vi "Event Handler.vi"(8 "error in (no error)":errorcluster, 11 "Data Grid in":refnum<class "Data Grid.lvclass">) -> (0 "error out":errorcluster, 3 "Data Grid out":refnum<class "Data Grid.lvclass">)   [LabVIEW 2013, in "Table Manager.lvlib" / "Data Grid.lvclass"]
uses:
  Data Grid.lvclass
  Data Grid.lvclass/Data Grid.ctl
  Table Manager.lvlib
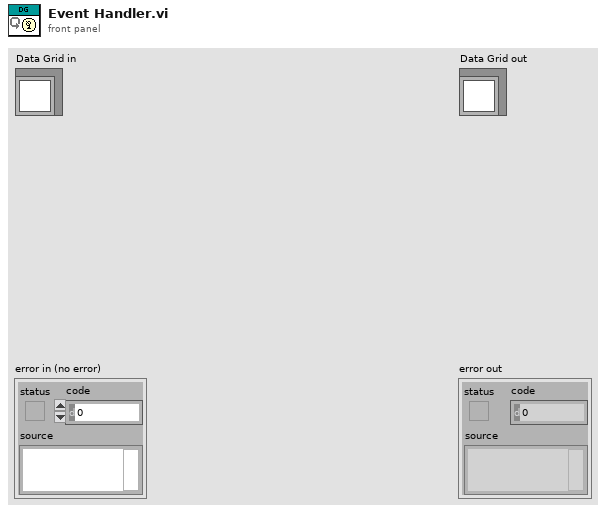
[diagram p1: front panel]
types:
  T1 = typedef "NISE_CEF_Node.lvclass/RefreshUIEvent.ctl" = refnum<user-event>
  T2 = cluster{"Data Grid":refnum<event-registration>, "Node Events":refnum<event-registration>}
  T3 = typedef "Table Manager.lvlib/Table Manager.lvclass/object ref.ctl" = cluster{"engine":refnum<data-value>, "Node Ref":refnum<data-value>}
  T4 = typedef "control module editor.lvclass/dialog output action.ctl" = enum16{"Tag Created", "Tag Selected", "Set Default", "disconnect"}
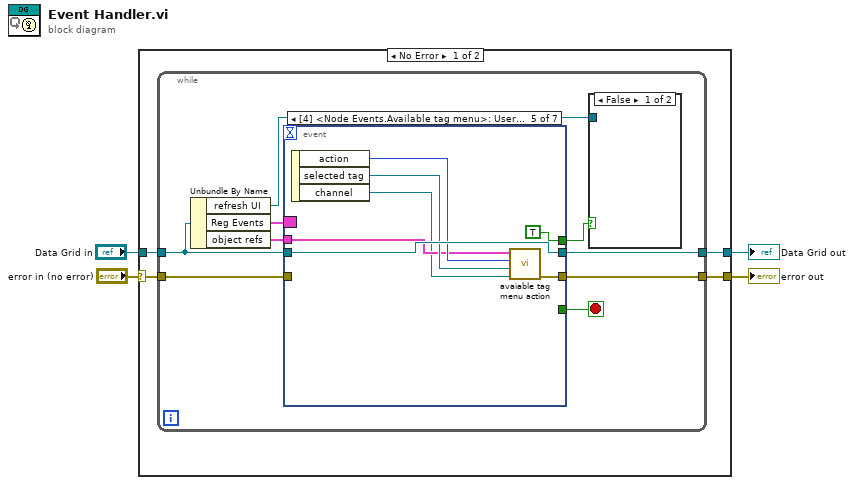
[diagram p0: block diagram]
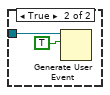
[diagram p2: hidden frame]
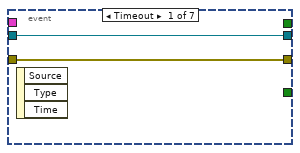
[diagram p3: hidden frame]
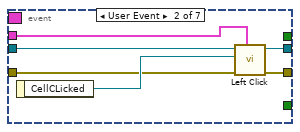
[diagram p4: hidden frame]
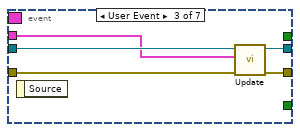
[diagram p5: hidden frame]
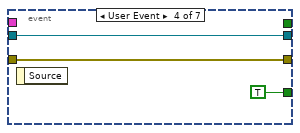
[diagram p6: hidden frame]
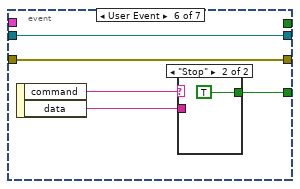
[diagram p7: hidden frame]
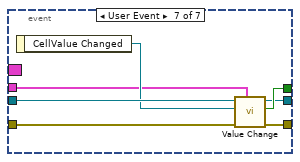
[diagram p9: hidden frame]
diagram:
  n1 = case shown="No Error" "error in (no error)" {
    selector: "error in (no error)" -> [w6 w56]
    tunnel: [w8 w57] -> w3
    tunnel: "Data Grid in" -> [w7 w57]
    tunnel: [w5 w56] -> w1
    frame No Error {
      n2 = while {
        tunnel: [w17] -> w8
        tunnel: w7 -> [w16]
        tunnel: w6 -> [w14]
        tunnel: [w13] -> w5
        stop <- w11 stop-if-true
        n3 = Unbundle By Name(w16) -> ("refresh UI"=w9:T1, "Reg Events"=w15:T2, "object refs"=w12:T3)
        n4 = event shown="[4] <Node Events.Available tag menu>: User Event" {
          selector: w15 -> [_ _ _ _ _ _ _]
          dyn-events: _ -> [_ _ _ _ _ _ _]
          timeout: _ -> [_ _ _ _ _ _ _]
          tunnel: [w21 w26 w31 w34 w42 w47 w53] -> w17
          tunnel: w16 -> [w21 w27 w32 w34 w42 w47 w54]
          tunnel: w14 -> [w20 w24 w30 w33 _ w46 w52]
          tunnel: [w20 w23 w29 w33 w37 w46 w51] -> w13
          tunnel: w12 -> [_ w22 w28 _ w39 _ w49]
          tunnel: [_ _ _ TRUE _ w43 _] -> w11
          tunnel: [_ _ _ _ TRUE _ w55] -> w10
          event Timeout {
            n5 = event-data() -> ()  [unwired: 1 in, 3 out]
          }
          event User Event {
            n6 = event-data() -> ("CellCLicked"=w25:refnum<class "Abstract EVENT.lvclass">)  [unwired: 1 in]
            n7 = call-dynamic "Left Click.vi"("object refs"=w22, "error in (no error)"=w24, "Event data"=w25, "Data Grid in"=w27) -> ("error out"=w23:errorcluster, "Data Grid out"=w26:refnum<class "Data Grid.lvclass">)  [unwired: 5 in, 1 out]
          }
          event User Event {
            n8 = event-data() -> ()  [unwired: 1 in, 1 out]
            n9 = call-dynamic "Update.vi"("error in"=w30, "object ref in"=w28, "Data Grid in"=w32) -> ("error out"=w29:errorcluster, "Data Grid out"=w31:refnum<class "Data Grid.lvclass">)  [unwired: 6 in, 1 out]
          }
          event User Event {
            n10 = event-data() -> ()  [unwired: 1 in, 1 out]
          }
          event User Event {
            n11 = event-data() -> ("action"=w40:T4, "selected tag"=w41:refnum<class "tag descriptor.lvclass">, "channel"=w38:refnum<class "TBM channel.lvclass">)  [unwired: 1 in]
            n12 = call "avaiable tag menu action.vi"("channel"=w38, "selected tag"=w41, "action"=w40, "object ref"=w39) -> ("error out"=w37:errorcluster)  [unwired: 6 in, 1 out]
          }
          event User Event {
            n13 = event-data() -> ("command"=w45:string, "data"=w44:string)  [unwired: 1 in]
            n14 = case shown="\"Stop\"" w45 {
              tunnel: [_ TRUE] -> w43
              tunnel: w44 -> [_ _]
              frame Default {
              }
              frame "Stop" {
              }
            }
          }
          event User Event {
            n15 = event-data() -> ("CellValue Changed"=w50:refnum<class "Abstract EVENT.lvclass">)  [unwired: 1 in]
            n16 = call-dynamic "Value Change.vi"("objects"=w49, "error in"=w52, "EVENT"=w50, "Data Grid in"=w54) -> ("error out"=w51:errorcluster, "Update?"=w55:bool, "Data Grid out"=w53:refnum<class "Data Grid.lvclass">)  [unwired: 5 in]
          }
        }
        n17 = case shown="False" w10 {
          tunnel: w9 -> [_ w18]
          frame False {
          }
          frame True {
            n18 = Generate User Event(user event=w18, event data cluster=TRUE ("event data")) -> ()  [unwired: 2 in, 2 out]
          }
        }
      }
    }
    frame Error {
    }
  }
  "error out" <- w1
  "Data Grid out" <- w3
